vi "PC_read_counts_in_buffer_or_not.vi"(9 "Actual Depth":u32, 10 "Elements Remaining":u32, 11 "Streaming Parameters":T1) -> (3 "Boolean":bool)   [LabVIEW 2020]
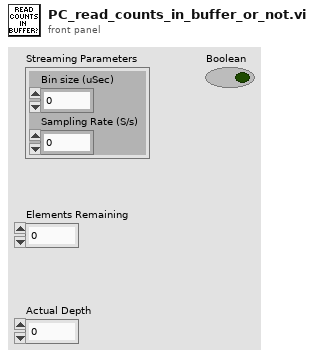
[diagram p1: front panel]
types:
  T1 = cluster{"Bin size (uSec)":u32, "Sampling Rate (S/s)":u32}
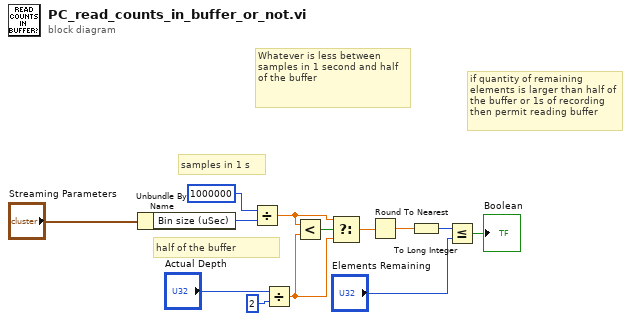
[diagram p0: block diagram]
diagram:
  # "if quantity of remaining elements is larger than half of the buffer or 1s of recording then permit reading buffer"
  # "Whatever is less between samples in 1 second and half of the buffer"
  # "half of the buffer"
  # "samples in 1 s"
  n1 = Unbundle By Name("Streaming Parameters") -> ("Bin size (uSec)"=w2:u32)
  n2 = Divide(x=u32 1000000, y=w2) -> (x/y=w7:dbl)
  n3 = Divide(x="Actual Depth", y=u32 2) -> (x/y=w8:dbl)
  n4 = Less?(x=w7, y=w8) -> (x < y?=w6:bool)
  n5 = Select(t=w7, s=w6, f=w8) -> (s? t:f=w9:dbl)
  n6 = Round To Nearest(number=w9) -> (nearest integer value=w10:dbl)
  n7 = To Long Integer(number=w10) -> (32bit integer=w11:i32)
  n8 = Less Or Equal?(x=w11, y="Elements Remaining") -> (x <= y?=→"Boolean":bool)
